vi "Load All Components.vi"(8 "error in (no error)":errorcluster, 11 "Component Loader in":refnum<class "Component Loader.lvclass">) -> (0 "error out":errorcluster, 2 "Components":refnum<class "Component.lvclass">[](array[class]), 3 "Component Loader out":refnum<class "Component Loader.lvclass">)   [LabVIEW 2017, in "DSF Core.lvlib" / "Component Loader.lvclass"]
uses:
  Component Loader.lvclass
  Component/Component.lvclass
  Component Loader.lvclass/Component Loader.ctl
  Component/Component.lvclass/Component.ctl
  Component/Default Buffer Converter/Create.vi
  Component/Default Buffer Converter/Default Buffer Converter Component.lvclass
  C:/Git/niveristand-data-sharing-framework-custom-device/Core/Classes/Component/Component.lvclass
  Component User Interface/Find.vi
  Component Configuration/Find.vi
  Components/Buffer Converters/DSF Type Converter/Default Buffer Converter.lvclass
  Components/Buffer Converters/DSF Type Converter/User Interfaces/Default Buffer Converter User Interfaces.lvclass
  Components/Buffer Converters/DSF Type Converter/Configurations/Default Buffer Converter Configurations.lvclass
  DSF Core.lvlib
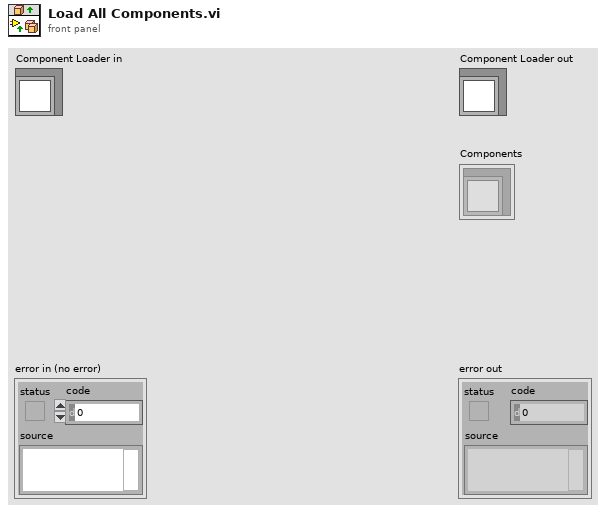
[diagram p1: front panel]
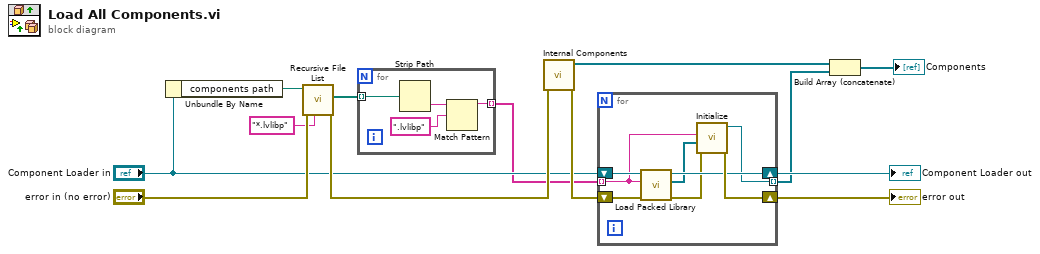
[diagram p0: block diagram]
diagram:
  n1 = Unbundle By Name("Component Loader in") -> ("components path"=w7:path)
  n2 = call <vilib>:"Recursive File List.vi"("pattern"="*.lvlibp", "error in (no error)"="error in (no error)", "Folder Path"=w7) -> ("error out"=w12:errorcluster, "All Files in Dir"=w6:path[])  [unwired: 4 in, 3 out]
  n3 = for {
    tunnel: w6 -> [w17] mode=indexing
    tunnel: [w14] -> w4 mode=indexing
    n4 = Strip Path(path=w17) -> (name=w16:string)  [unwired: 1 out]
    n5 = Match Pattern(string=w16, regular expression=".lvlibp") -> (before substring=w14:string)  [unwired: 1 in, 3 out]
  }
  n6 = call "Internal Components.vi"("error in (no error)"=w12) -> ("error out"=w9:errorcluster, "Components"=w3:refnum<class "Component.lvclass">[])  [unwired: 9 in]
  n7 = for {
    shift-right: [w22] -> w11
    shift-left: "Component Loader in" -> [w25]
    shift-right: [w23] -> w10
    shift-left: w9 -> [w24]
    tunnel: w4 -> [w18] mode=indexing
    tunnel: [w21] -> w2 mode=indexing
    n8 = call "Load Packed Library.vi"("error in (no error)"=w24, "packed library name"=w18, "Component Loader in"=w25) -> ("error out"=w20:errorcluster, "objects"=w19:refnum<class>[], "Component Loader out"=w22:refnum<class "Component Loader.lvclass">)  [unwired: 6 in]
    n9 = call "Initialize.vi"("error in (no error)"=w20, "objects"=w19, "name"=w18) -> ("error out"=w23:errorcluster, "Component out"=w21:refnum<class "Component.lvclass">)  [unwired: 7 in]
  }
  "error out" <- w10
  "Component Loader out" <- w11
  n10 = Build Array (concatenate)(w3, w2) -> (→"Components":refnum<class "Component.lvclass">[])
